vi "Replace Item in Array (CTL).vi"(8 "error in":errorcluster, 10 "Array Item Replacement Params":T1, 11 "Original VI":path=path "C:/Users/OneEd/OneDrive/Desktop/MicroPort Job/CTDB/src/db_script/DB Select Template.vi") -> (0 "error out":errorcluster, 3 "Save as out":path=path "C:/Users/OneEd/OneDrive/Desktop/MicroPort Job/CTDB/src/db_script/DB Select Template.vi")   [LabVIEW 2021, in "EDT VI Script.lvlib"]
uses:
  EDT VI Script.lvlib
  Array Item Replacement Param (CTL).ctl
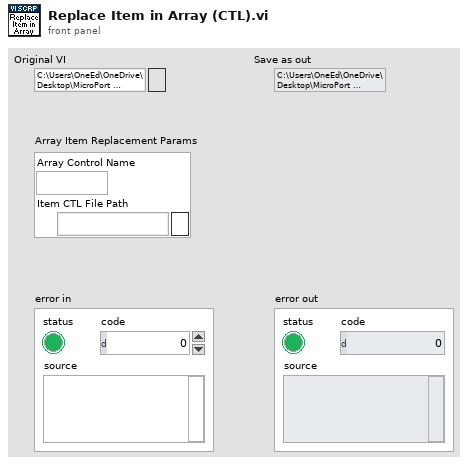
[diagram p1: front panel]
types:
  T1 = typedef "EDT VI Script.lvlib/Array Item Replacement Param (CTL).ctl" = cluster{"Array Control Name":string, "Item CTL File Path":path}
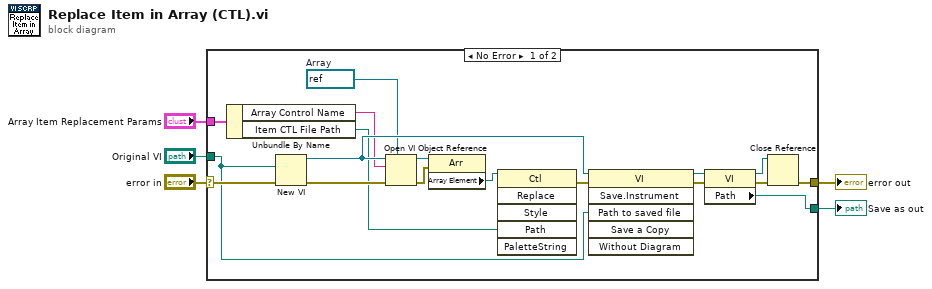
[diagram p0: block diagram]
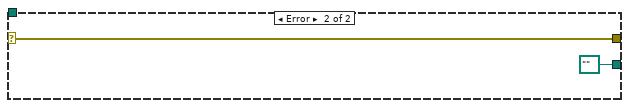
[diagram p2: hidden frame]
diagram:
  n1 = case shown="No Error" "error in" {
    selector: "error in" -> [w23 w25]
    tunnel: [w20 w25] -> w4
    tunnel: "Original VI" -> [w13 _]
    tunnel: "Array Item Replacement Params" -> [w21 _]
    tunnel: [w16 path "" ("Path")] -> w1
    frame No Error {
      w10 = refnum<vi> refnum  # Array
      n2 = Unbundle By Name(w21) -> ("Array Control Name"=w12:string, "Item CTL File Path"=w11:path)
      n3 = New VI(8:w23, 10:w13) -> (0:w22:errorcluster, 3:w19:refnum<vi>)  [unwired: 5 in]
      n4 = Open VI Object Reference(7:w10, 8:w22, 10:w12, 11:w19) -> (0:w8:errorcluster, 3:w9:refnum<vi>)
      n5 = property class="Arr"(reference=w9, error in=w8) -> ("Array Element"=w7:refnum<vi>)  [unwired: 2 out]
      n6 = invoke on="Invoke Node" class="Ctl" method="Replace"(reference=w7, "Path"=w11) -> (error out=w6:errorcluster)  [unwired: 4 in, 5 out]
      n7 = invoke class="VI" method="Save.Instrument"(reference=w19, error in=w6, "Path to saved file"=w13) -> (reference out=w15:refnum<vi>, error out=w14:errorcluster)  [unwired: 3 in, 4 out]
      n8 = property class="VI"(reference=w15, error in=w14) -> (reference out=w18:refnum<vi>, error out=w17:errorcluster, "Path"=w16:path)
      n9 = Close Reference(reference=w18, error in (no error)=w17) -> (error out=w20:errorcluster)
    }
    frame Error {
    }
  }
  "error out" <- w4
  "Save as out" <- w1
